vi "Read message_data.vi"(8 "error in (no error)":errorcluster, 11 "SOAP Data in":refnum<class "SOAP Data.lvclass">) -> (0 "error out":errorcluster, 2 "message_data":refnum<data-value>, 3 "SOAP Data out":refnum<class "SOAP Data.lvclass">)   [LabVIEW 2016, in "Controller.lvlib" / "SOAP Data.lvclass"]
uses:
  SOAP Data.lvclass
  SOAP Data.lvclass/SOAP Data.ctl
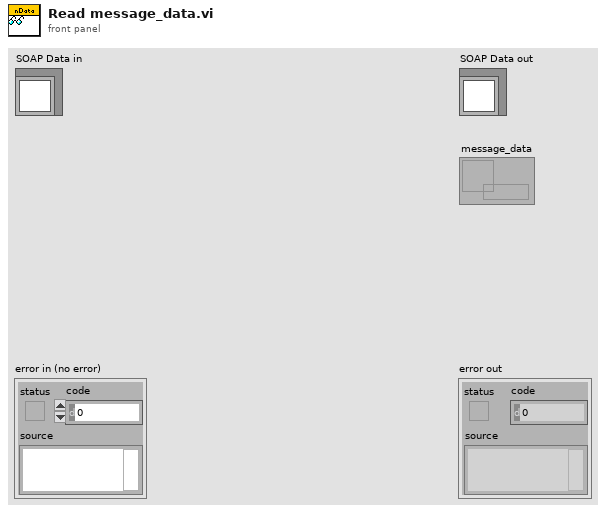
[diagram p1: front panel]
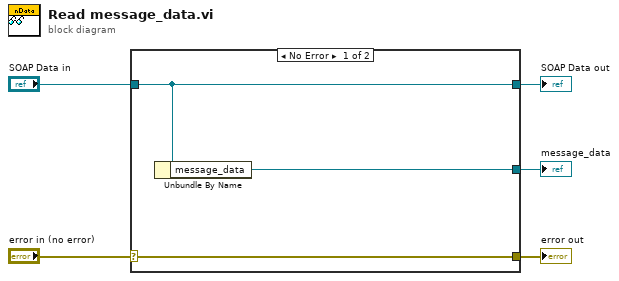
[diagram p0: block diagram]
diagram:
  n1 = case shown="No Error" "error in (no error)" {
    selector: "error in (no error)" -> [w8 w9]
    tunnel: [w8 w9] -> w4
    tunnel: [w7 w10] -> w2
    tunnel: "SOAP Data in" -> [w7 w10]
    tunnel: [w6 _] -> w1
    frame No Error {
      n2 = Unbundle By Name(w7) -> ("message_data"=w6:refnum<data-value>)
    }
    frame Error {
    }
  }
  "error out" <- w4
  "SOAP Data out" <- w2
  "message_data" <- w1
